vi "GDFdisplayEventTable.vi"(7 "Select Event Type":refnum<vi>, 8 "error in (no error)":errorcluster, 9 "Samplerate":dbl, 10 "Array of Events in":T1[](array[typedef]), 11 "Multicolumn Listbox in":refnum<vi>) -> (0 "error out":errorcluster)   [LabVIEW 2016, in "GDF File Reader.lvlib"]
uses:
  GDF File Reader.lvlib
  EventDataType.ctl
panel:
  # "This VI is a part of BCI Design library, http://www.ru-bci.org \nCopyright © 2020, Sotnikov Peter, All rights reserved. License: CC BY-NC 4.0"
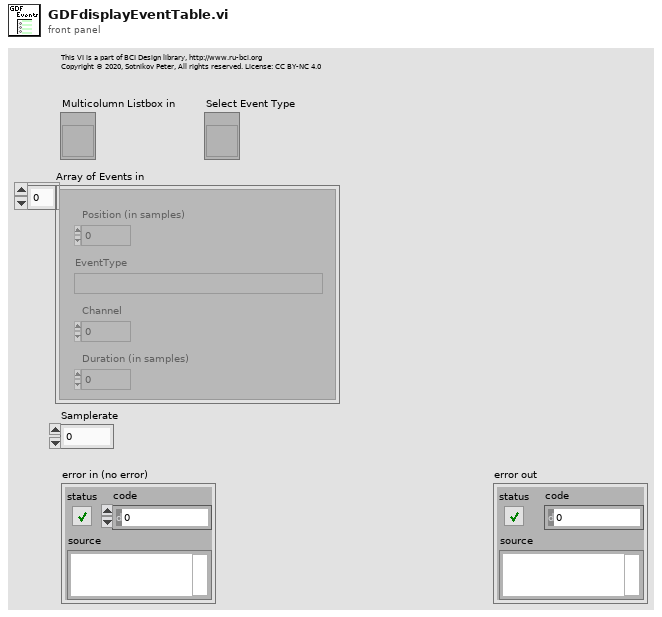
[diagram p1: front panel]
types:
  T1 = typedef "GDF File Reader.lvlib/EventDataType.ctl" = cluster{"Position (in samples)":u32, "EventType":string, "Channel":u16, "Duration (in samples)":u32}
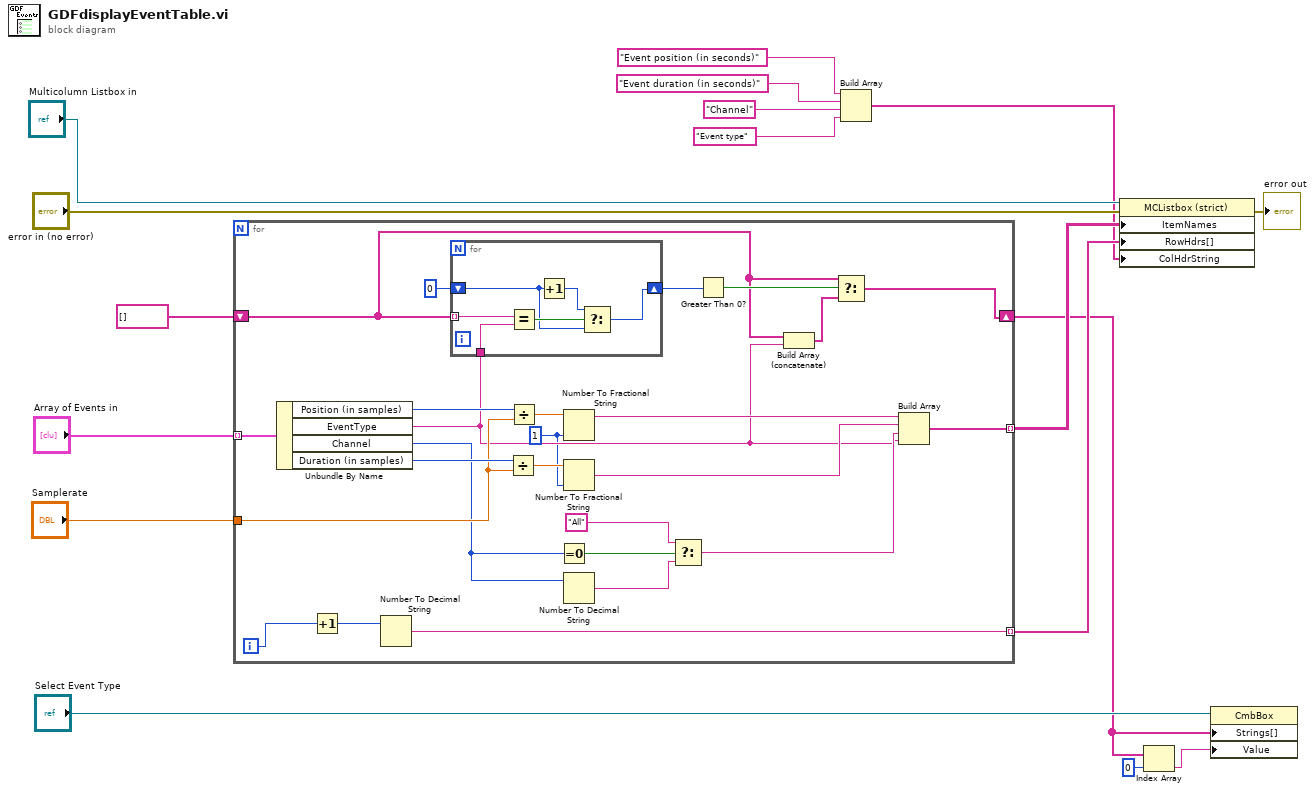
[diagram p0: block diagram]
diagram:
  n1 = for {
    tunnel: "Array of Events in" -> [w42] mode=indexing
    tunnel: [w39] -> w13 mode=indexing
    tunnel: "Samplerate" -> [w36]
    tunnel: [w26] -> w14 mode=indexing
    shift-right: [w19] -> w4
    shift-left: string[] [] -> [w22]
    i -> [w41]
    w18 = i16 1 ("precision (6)")
    n2 = Unbundle By Name(w42) -> ("Position (in samples)"=w38:u32, "EventType"=w21:string, "Channel"=w33:u16, "Duration (in samples)"=w37:u32)
    n3 = Increment(x=w41) -> (x+1=w40:i32)
    n4 = Number To Decimal String(number=w40) -> (decimal integer string=w39:string)  [unwired: 1 in]
    n5 = for {
      tunnel: w22 -> [w48] mode=indexing
      tunnel: w21 -> [w47]
      shift-right: [w43] -> w24
      shift-left: 0 -> [w44]
      n6 = Equal?(x=w48, y=w47) -> (x = y?=w46:bool)
      n7 = Increment(x=w44) -> (x+1=w45:i32)
      n8 = Select(t=w45, s=w46, f=w44) -> (s? t:f=w43:i32)
    }
    n9 = Divide(x=w37, y=w36) -> (x/y=w35:dbl)
    n10 = Divide(x=w38, y=w36) -> (x/y=w34:dbl)
    n11 = Equal To 0?(x=w33) -> (x = 0?=w32:bool)
    n12 = Number To Fractional String(number=w34, precision (6)=w18) -> (F-format string=w29:string)  [unwired: 2 in]
    n13 = Number To Fractional String(number=w35, precision (6)=w18) -> (F-format string=w28:string)  [unwired: 2 in]
    n14 = Number To Decimal String(number=w33) -> (decimal integer string=w31:string)  [unwired: 1 in]
    n15 = Select(t="All", s=w32, f=w31) -> (s? t:f=w27:string)
    n16 = Greater Than 0?(x=w24) -> (x > 0?=w23:bool)
    n17 = Build Array (concatenate)(w22, w21) -> (w20:string[])
    n18 = Select(t=w22, s=w23, f=w20) -> (s? t:f=w19:string[])
    n19 = Build Array(w29, w28, w27, w21) -> (w26:string[])
  }
  n20 = Build Array("Event position (in seconds)", "Event duration (in seconds)", "Channel", "Event type") -> (w7:string[])
  n21 = property class="MCListbox (strict)"(reference="Multicolumn Listbox in", error in="error in (no error)", "ItemNames"=w14, "RowHdrs[]"=w13, "ColHdrString"=w7) -> (error out=→"error out":errorcluster)  [unwired: 1 out]
  n22 = Index Array(array=w4, index=0) -> (element=w2:string)
  n23 = property class="CmbBox"(reference="Select Event Type", "Strings[]"=w4, "Value"=w2) -> ()  [unwired: 1 in, 2 out]
